vi "FEED_Update_Cycle_Status.vi"(7 "Enum":enum16{"FEED", "LOADED"}(ring)=enum."LOADED", 8 "error in (no error)":errorcluster, 10 "Door No":i32, 11 "?":T1) -> (0 "error out":errorcluster, 2 "?":T1, 3 "output array":string[][](array[string]))   [LabVIEW 2017]
uses:
  Controls/Feed_Cyc_Data.ctl
  <vilib>/Utility/file.llb/Read Delimited Spreadsheet (string).vi
  <vilib>/Utility/file.llb/Write Delimited Spreadsheet (string).vi
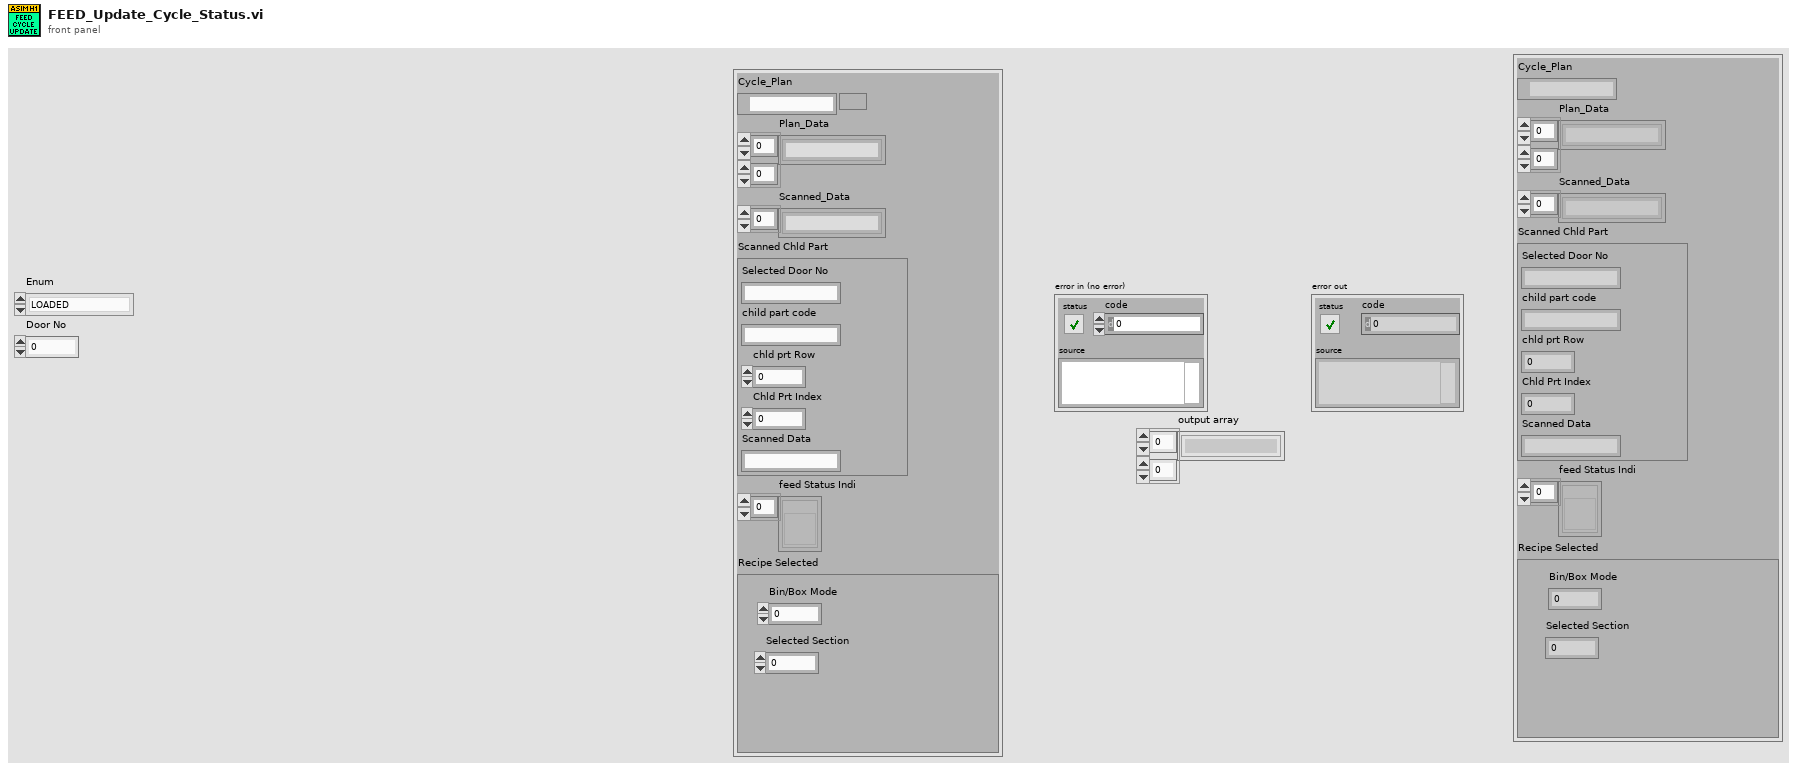
[diagram p1: front panel]
types:
  T1 = typedef "Feed_Cyc_Data.ctl" = cluster{"Cycle_Plan":path, "Plan_Data":string[][], "Scanned_Data":string[], "Scanned Chld Part":cluster{"Selected Door No":string, "child part code":string, "chld prt Row":i32, "Chld Prt Index":i32, "Scanned Data":string}, "feed Status Indi":refnum<vi>[], "Recipe Selected":cluster{"Bin/Box Mode":i32, "Selected Section":i32}}
  T2 = cluster{"Selected Door No":string, "child part code":string, "chld prt Row":i32, "Chld Prt Index":i32, "Scanned Data":string}
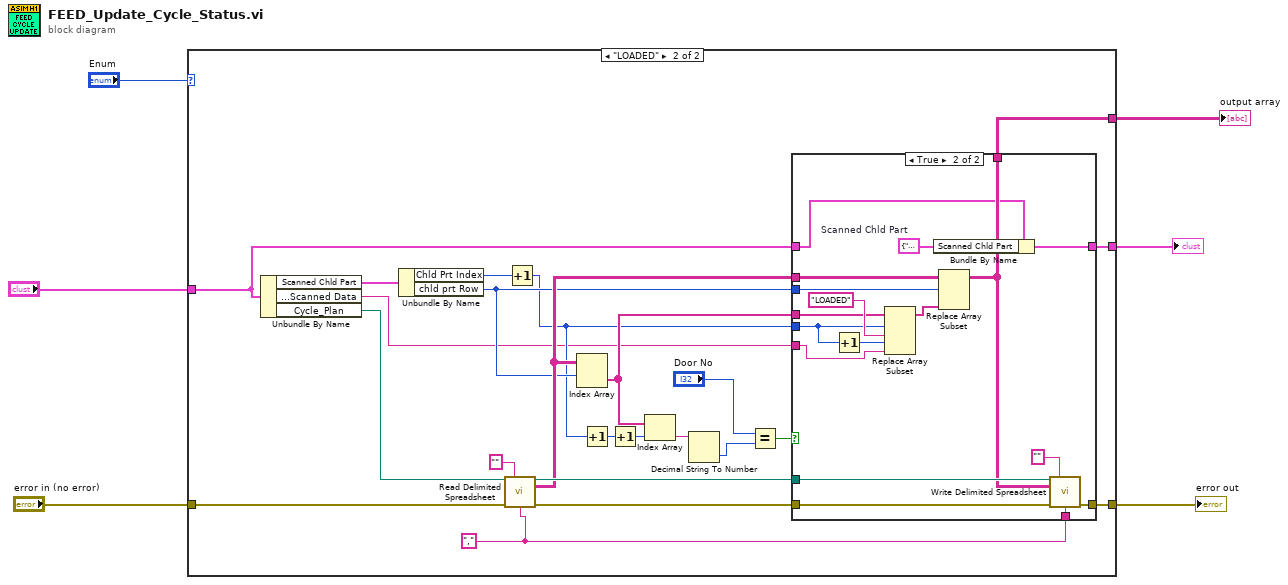
[diagram p0: block diagram]
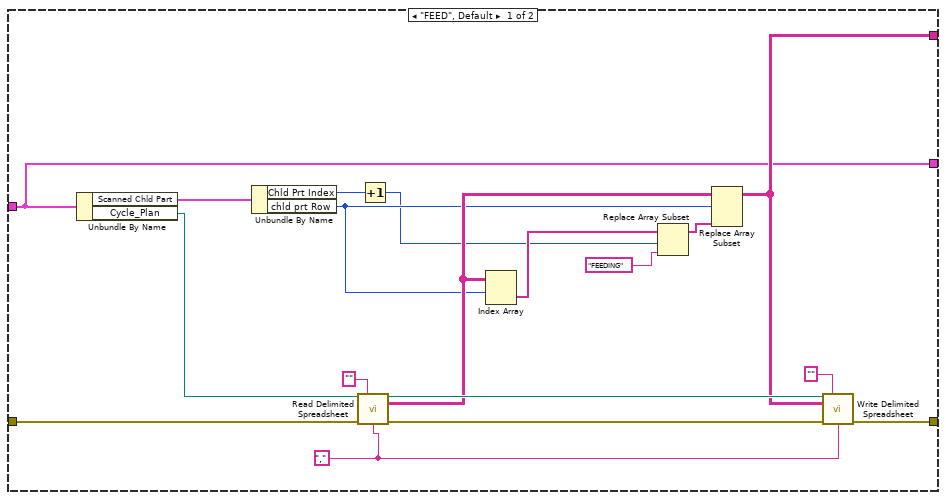
[diagram p2: hidden frame]
diagram:
  n1 = case shown="\"LOADED\"" "Enum" {
    tunnel: "?" -> [w7 w28]
    tunnel: "error in (no error)" -> [w21 w45]
    tunnel: [w20 w44] -> w4
    tunnel: [w11 w40] -> w3
    tunnel: [w7 w27] -> w1
    frame "FEED", Default {
      w10 = ","
      n2 = Unbundle By Name(w7) -> ("Scanned Chld Part"=w19:T2, "Cycle_Plan"=w23:path)
      n3 = Unbundle By Name(w19) -> ("Chld Prt Index"=w15:i32, "chld prt Row"=w17:i32)
      n4 = call-poly <vilib>:"Read Delimited Spreadsheet.vi"("file path (dialog if empty)"=w23, "format (%s)"="", "error in (no error)"=w21, "delimiter (\\t)"=w10) -> ("new file path (Not A Path if cancelled)"=w22:path, "all rows"=w18:string[][], "error out"=w24:errorcluster)  [unwired: 6 in, 3 out]
      n5 = Increment(x=w15) -> (x+1=w14:i32)
      n6 = Index Array(array=w18, index (row)=w17) -> (element=w16:string[])  [unwired: 1 in]
      n7 = Replace Array Subset(array=w16, new element="FEEDING", index=w14) -> (w12:string[])
      n8 = Replace Array Subset(array=w18, new element=w12, index (row)=w17) -> (w11:string[][])  [unwired: 1 in]
      n9 = call-poly <vilib>:"Write Delimited Spreadsheet.vi"("file path (dialog if empty)"=w22, "format (%s)"="", "2D data"=w11, "error in (no error)"=w24, "delimiter (\\t)"=w10) -> ("error out"=w20:errorcluster)  [unwired: 9 in, 1 out]
    }
    frame "LOADED" {
      w39 = ","
      n10 = Unbundle By Name(w28) -> ("Scanned Chld Part"=w43:T2, "Scanned Chld Part.Scanned Data"=w26:string, "Cycle_Plan"=w25:path)
      n11 = Unbundle By Name(w43) -> ("Chld Prt Index"=w41:i32, "chld prt Row"=w37:i32)
      n12 = call-poly <vilib>:"Read Delimited Spreadsheet.vi"("file path (dialog if empty)"=w25, "format (%s)"="", "error in (no error)"=w45, "delimiter (\\t)"=w39) -> ("new file path (Not A Path if cancelled)"=w46:path, "all rows"=w42:string[][], "error out"=w47:errorcluster)  [unwired: 6 in, 3 out]
      n13 = Increment(x=w41) -> (x+1=w35:i32)
      n14 = Index Array(array=w42, index (row)=w37) -> (element=w36:string[])  [unwired: 1 in]
      n15 = Increment(x=w35) -> (x+1=w33:i32)
      n16 = Increment(x=w33) -> (x+1=w34:i32)
      n17 = Index Array(array=w36, index=w34) -> (element=w32:string)
      n18 = Decimal String To Number(string=w32) -> (number=w31:i32)  [unwired: 2 in, 1 out]
      n19 = Equal?(x="Door No", y=w31) -> (x = y?=w29:bool)
      n20 = case shown="True" w29 {
        tunnel: w47 -> [w49 w67]
        tunnel: w46 -> [_ w66]
        tunnel: [w49 w65] -> w44
        tunnel: w42 -> [w50 w64]
        tunnel: [w50 w61] -> w40
        tunnel: w39 -> [_ w60]
        tunnel: w37 -> [_ w59]
        tunnel: w36 -> [_ w58]
        tunnel: w35 -> [_ w52]
        tunnel: w28 -> [w48 w56]
        tunnel: [w48 w55] -> w27
        tunnel: w26 -> [_ w51]
        frame False {
        }
        frame True {
          w54 = T2 {"Selected Door No"="", "child part code"="", "chld prt Row"=0, "Chld Prt Index"=0, "Scanned Data"=""}  # Scanned Chld Part
          n21 = Increment(x=w52) -> (x+1=w53:i32)
          n22 = Replace Array Subset(array=w58, new element #1="LOADED", index #1=w52, new element #2=w51, index #2=w53) -> (w62:string[])
          n23 = Bundle By Name(cluster=w56, "Scanned Chld Part"=w54) -> (w55:T1)
          n24 = Replace Array Subset(array=w64, new element=w62, index (row)=w59) -> (w61:string[][])  [unwired: 1 in]
          n25 = call-poly <vilib>:"Write Delimited Spreadsheet.vi"("file path (dialog if empty)"=w66, "format (%s)"="", "2D data"=w61, "error in (no error)"=w67, "delimiter (\\t)"=w60) -> ("error out"=w65:errorcluster)  [unwired: 9 in, 1 out]
        }
      }
    }
  }
  "error out" <- w4
  "output array" <- w3
  "?" <- w1
